vi "BRig_dataTrial_sTrial_start.vi"() -> (2 "output_sTrial_start":i32)   [LabVIEW 2014]
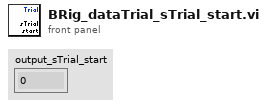
[diagram p1: front panel]
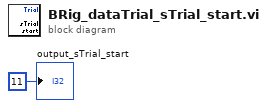
[diagram p0: block diagram]
diagram:
  "output_sTrial_start" <- 11 ("output_iBlock")
